vi "Panel Global Data.vi"(7 "Method (Read All)":T2, 8 "error in (no error)":errorcluster, 10 "Panel Data In":T1, 11 "Panel VI Name":string) -> (0 "error out":errorcluster, 2 "Panel Data Out":T1, 3 "All Panel Data":T1[](array[typedef]), 5 "Panel VI Names":string[](array[string]))   [LabVIEW 2011]
doc: "This is an example VIG or Functional global that can be used as a template. Replace the Variant Data In, and Variant Data Out with the data type you want, or use a Variant Repository."
uses:
  Panel Global Methods.ctl
  Panel Data.ctl
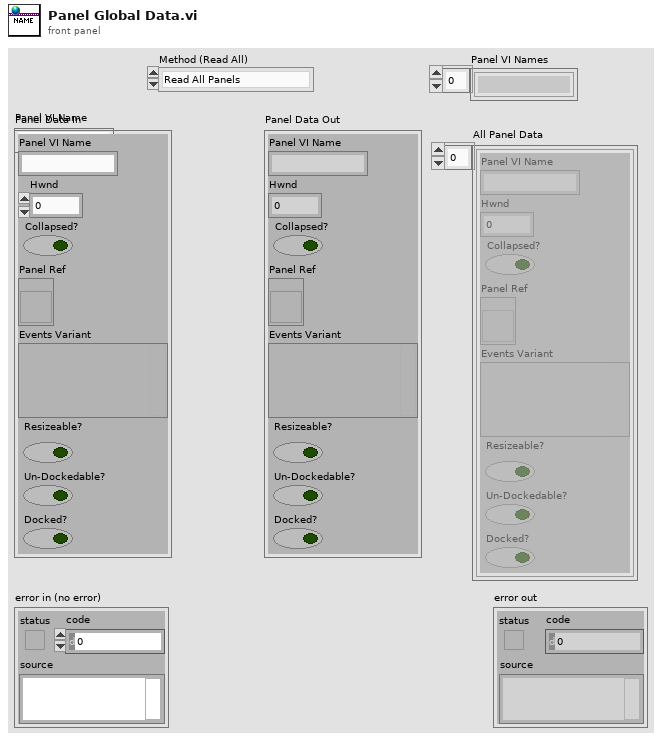
[diagram p1: front panel]
types:
  T1 = typedef "Panel Data.ctl" = cluster{"Panel VI Name":string, "Hwnd":u32, "Collapsed?":bool, "Panel Ref":refnum<vi>, "Events Variant":variant, "Resizeable?":bool, "Un-Dockedable?":bool, "Docked?":bool}
  T2 = typedef "Panel Global Methods.ctl" = enum16{"Read All Panels", "Read Panel Data", "Write Panel Data"}
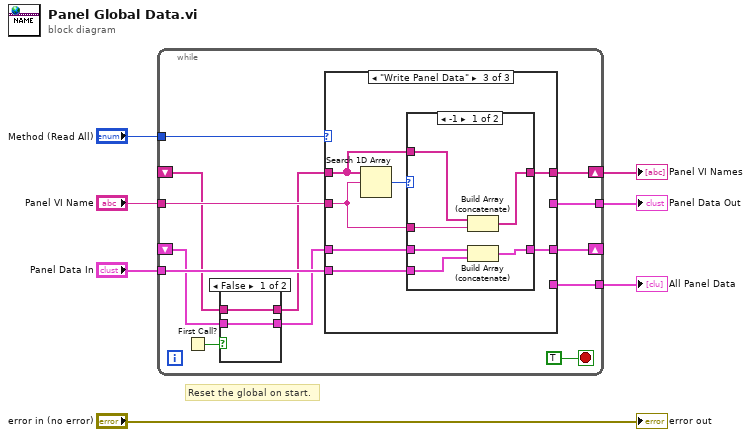
[diagram p0: block diagram]
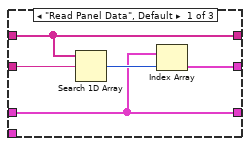
[diagram p3: hidden frame]
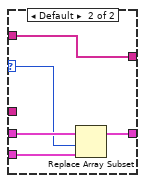
[diagram p5: hidden frame]
diagram:
  # "Reset the global on start."
  n1 = while {
    tunnel: "Method (Read All)" -> [w20]
    tunnel: "Panel VI Name" -> [w19]
    shift-right: [w18] -> w1
    shift-left: _ -> [w11]
    tunnel: "Panel Data In" -> [w16]
    shift-right: [w15] -> _
    shift-left: _ -> [w9]
    tunnel: [w14] -> w3
    tunnel: [w13] -> w2
    stop <- TRUE stop-if-true
    n2 = First Call?() -> (First Call?: T/F=w12:bool)
    n3 = case shown="False" w12 {
      tunnel: w11 -> [w22 _]
      tunnel: [w22 _] -> w10
      tunnel: w9 -> [w21 _]
      tunnel: [w21 _] -> w8
      frame False {
      }
      frame True {
      }
    }
    n4 = case shown="\"Write Panel Data\"" w20 {
      tunnel: w19 -> [w26 _ w35]
      tunnel: [w27 w29 w34] -> w18
      tunnel: w10 -> [w27 w29 w33]
      tunnel: w16 -> [_ _ w32]
      tunnel: [w24 w28 w31] -> w15
      tunnel: w8 -> [w24 w28 w30]
      tunnel: [w23 _ _] -> w14
      tunnel: [_ w28 _] -> w13
      frame "Read Panel Data", Default {
        n5 = Search 1D Array(1D array=w27, element=w26) -> (index of element=w25:i32)  [unwired: 1 in]
        n6 = Index Array(array=w24, index=w25) -> (element=w23:T1)
      }
      frame "Read All Panels" {
      }
      frame "Write Panel Data" {
        n7 = Search 1D Array(1D array=w33, element=w35) -> (index of element=w36:i32)  [unwired: 1 in]
        n8 = case shown="-1" w36 {
          selector: w36 -> [_ w43]
          tunnel: w35 -> [w42 _]
          tunnel: [w41 w47] -> w34
          tunnel: w33 -> [w40 w47]
          tunnel: w32 -> [w39 w44]
          tunnel: [w38 w46] -> w31
          tunnel: w30 -> [w37 w45]
          frame -1 {
            n9 = Build Array (concatenate)(w40, w42) -> (w41:string[])
            n10 = Build Array (concatenate)(w37, w39) -> (w38:T1[])
          }
          frame Default {
            n11 = Replace Array Subset(array=w45, new element=w44, index=w43) -> (w46:T1[])
          }
        }
      }
    }
  }
  "All Panel Data" <- w2
  "Panel Data Out" <- w3
  "Panel VI Names" <- w1
  "error out" <- "error in (no error)"
